vi "SDCP - Standard Message Frame Parameters - FGV.vi"(0 "SMF Parameters descriptors in":T1[](array[typedef]), 1 "Parameter file path":path, 2 "FID":i32, 3 "error in (no error)":errorcluster, 4 "Command":T2=enum."Read descriptors") -> (5 "SMF Parameters descriptors out":T1[](array[typedef]), 8 "error out":errorcluster)   [LabVIEW 2020]
uses:
  Typedefs/SDCP - SMF parameter descriptors.ctl
  Typedefs/SDCP - Standard Message Frame Parameters - FGV - commands.ctl
  Typedefs/SDCP - Standard Message Frames FGV - Commands.ctl
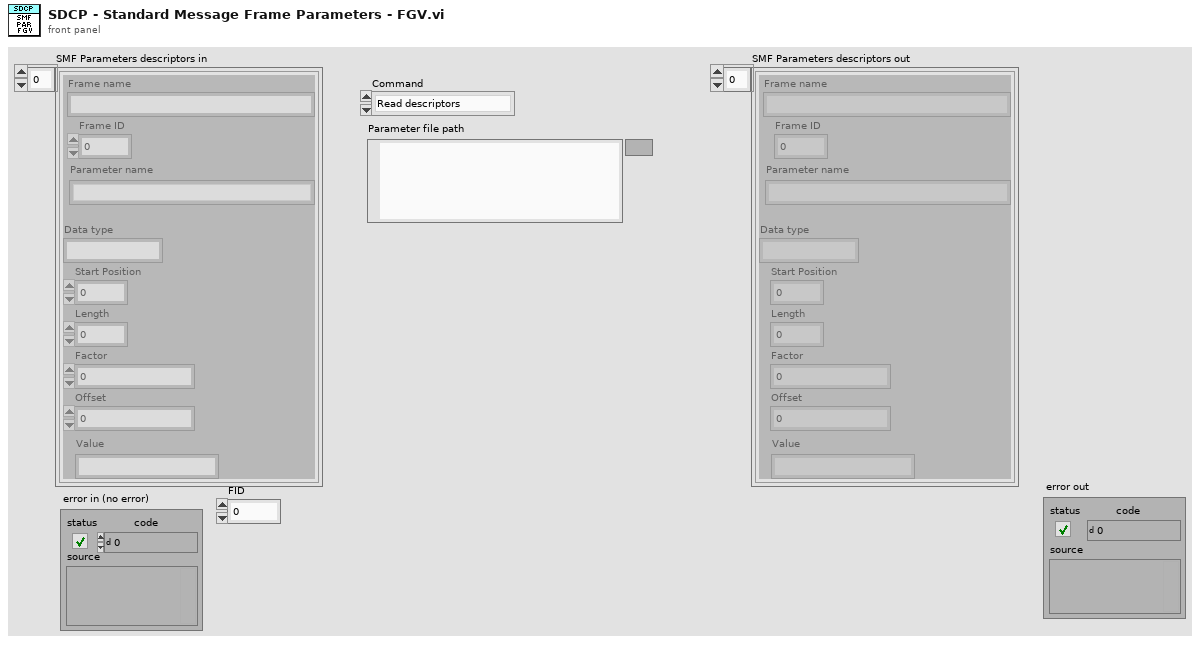
[diagram p1: front panel]
types:
  T1 = typedef "SDCP - SMF parameter descriptors.ctl" = cluster{"Frame name":string, "Frame ID":i32, "Data type":string, "Start Position":i32, "Length":i32, "Factor":dbl, "Offset":dbl, "Parameter name":string, "Value":string}
  T2 = typedef "SDCP - Standard Message Frame Parameters - FGV - commands.ctl" = enum16{"Write descriptors", "Read descriptors", "Read values", "Load parameters from file", "Write values", "Read all descriptors"}
  T3 = typedef "SDCP - Standard Message Frames FGV - Commands.ctl" = enum16{"Reset", "Read", "Write", "Set Priority"}
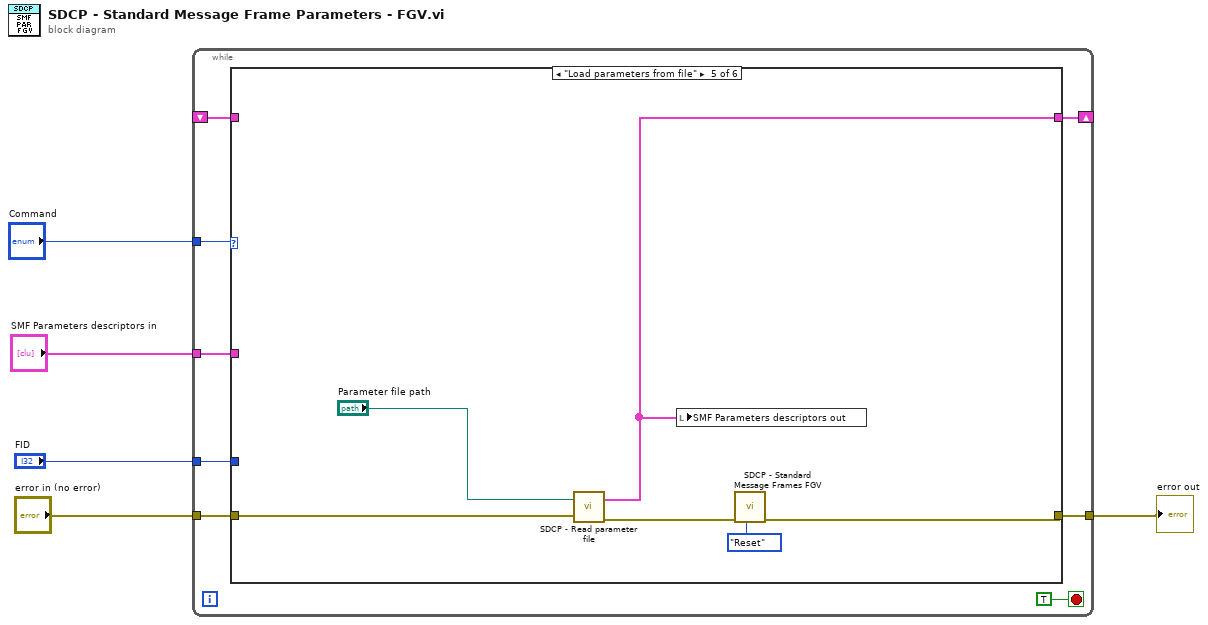
[diagram p0: block diagram]
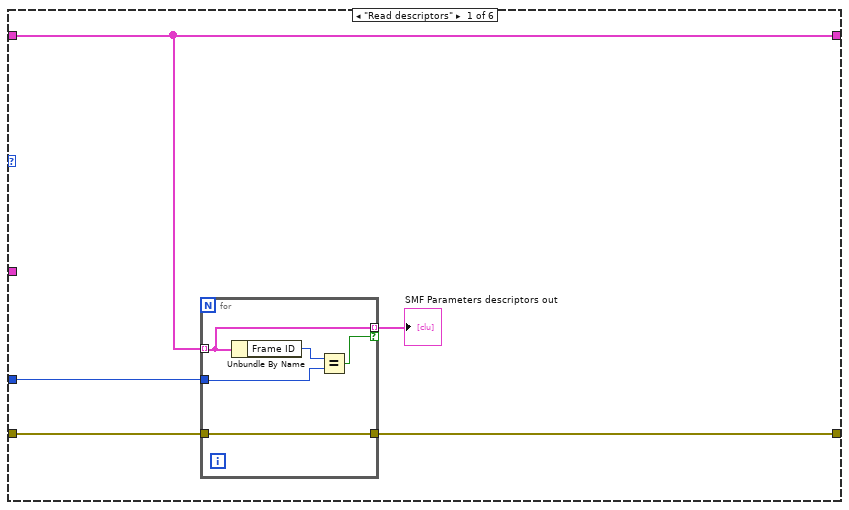
[diagram p2: hidden frame]
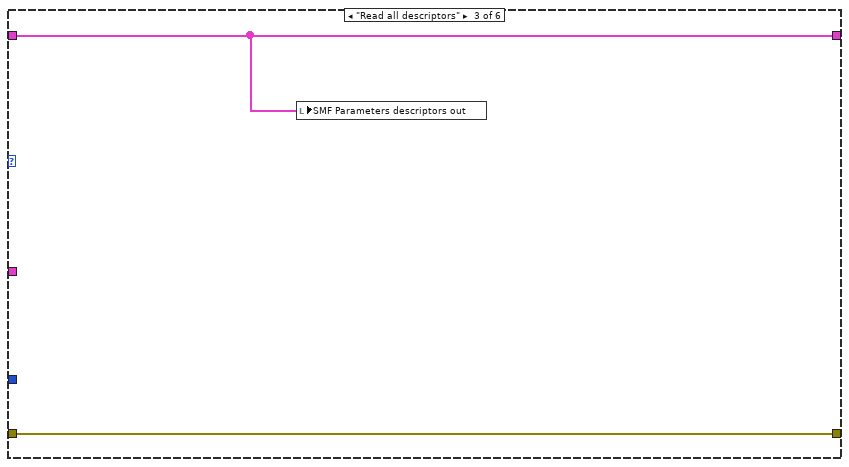
[diagram p4: hidden frame]
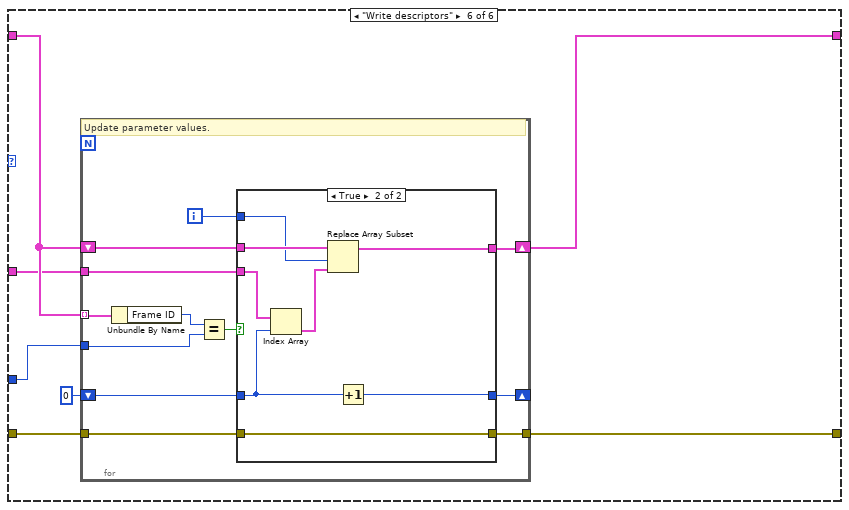
[diagram p6: hidden frame]
diagram:
  n1 = while {
    tunnel: "Command" -> [w12]
    tunnel: "FID" -> [w11]
    tunnel: "error in (no error)" -> [w10]
    tunnel: "SMF Parameters descriptors in" -> [w9]
    shift-right: [w8] -> _
    shift-left: _ -> [w6]
    tunnel: [w7] -> w1
    stop <- TRUE stop-if-true
    n2 = case shown="\"Load parameters from file\"" w12 {
      tunnel: w11 -> [w18 _ _ _ _ w41]
      tunnel: w10 -> [w17 w24 w27 w28 w35 w42]
      tunnel: w9 -> [_ _ _ _ _ w38]
      tunnel: [w15 w25 w26 w29 w33 w37] -> w8
      tunnel: [w16 w24 w27 w28 w31 w36] -> w7
      tunnel: w6 -> [w15 w25 w26 w29 _ w39]
      frame "Read descriptors" {
        n3 = for {
          tunnel: w15 -> [w20] mode=indexing
          tunnel: w18 -> [w23]
          tunnel: [w20] -> w14 mode=indexing if=w22
          tunnel: w17 -> [w21]
          tunnel: [w21] -> w16
          n4 = Unbundle By Name(w20) -> ("Frame ID"=w19:i32)
          n5 = Equal?(x=w19, y=w23) -> (x = y?=w22:bool)
        }
        "SMF Parameters descriptors out" <- w14
      }
      frame "Read values" {
      }
      frame "Read all descriptors" {
        n6 = local write "SMF Parameters descriptors out"(w26) -> ()
      }
      frame "Write values" {
      }
      frame "Load parameters from file" {
        n7 = call "SDCP - Read parameter file.vi"("error in (no error)"=w35, "Parameter file path"="Parameter file path") -> ("error out"=w32:errorcluster, "Parameter descriptors"=w33:T1[])
        n8 = local write "SMF Parameters descriptors out"(w33) -> ()
        n9 = call "SDCP - Standard Message Frames FGV.vi"("error in (no error)"=w32, "Command"=SDCP_-_Standard_Message_Frames_FGV_-_Commands."Reset") -> ("error out"=w31:errorcluster)  [unwired: 4 in, 2 out]
      }
      frame "Write descriptors" {
        n10 = for {
          tunnel: w39 -> [w53] mode=indexing
          tunnel: w41 -> [w54]
          tunnel: w42 -> [w51]
          tunnel: [w49] -> w36
          shift-right: [w47] -> _
          shift-left: 0 -> [w48]
          shift-right: [w45] -> w37
          shift-left: w39 -> [w46]
          tunnel: w38 -> [w44]
          i -> [w43]
          # "Update parameter values."
          n11 = Unbundle By Name(w53) -> ("Frame ID"=w52:i32)
          n12 = Equal?(x=w52, y=w54) -> (x = y?=w50:bool)
          n13 = case shown="True" w50 {
            tunnel: w51 -> [w57 w65]
            tunnel: [w57 w65] -> w49
            tunnel: w48 -> [w56 w61]
            tunnel: [w56 w60] -> w47
            tunnel: w46 -> [w55 w64]
            tunnel: [w55 w63] -> w45
            tunnel: w44 -> [_ w62]
            tunnel: w43 -> [_ w58]
            frame False {
            }
            frame True {
              n14 = Index Array(array=w62, index=w61) -> (element=w59:T1)
              n15 = Replace Array Subset(array=w64, new element=w59, index=w58) -> (w63:T1[])
              n16 = Increment(x=w61) -> (x+1=w60:i32)
            }
          }
        }
      }
    }
  }
  "error out" <- w1
